vi "ziModSetVector.vi"(8 "error in":errorcluster, 9 "VectorWave In":T2, 10 "Path":string, 11 "ModHandle In":T1 {"ModHandle" format="0x%08x"; "Conn" format="0x%08x"}) -> (0 "error out":errorcluster, 3 "ModHandle Out":T1 {"ModHandle" format="0x%08x"; "Conn" format="0x%08x"})   [LabVIEW 2009, in "Zurich Instruments LabOne.lvlib"]
uses:
  <instrlib>/Zurich Instruments LabOne/Zurich Instruments LabOne.lvlib
  <instrlib>/Zurich Instruments LabOne/Public/Data/ziTypeCoreVectorWave.ctl
  <instrlib>/Zurich Instruments LabOne/Public/Modules/ziTypeModHandle.ctl
  <instrlib>/Zurich Instruments LabOne/Private/ziLV32.dll
panel:
  out "VectorWave Out":T2
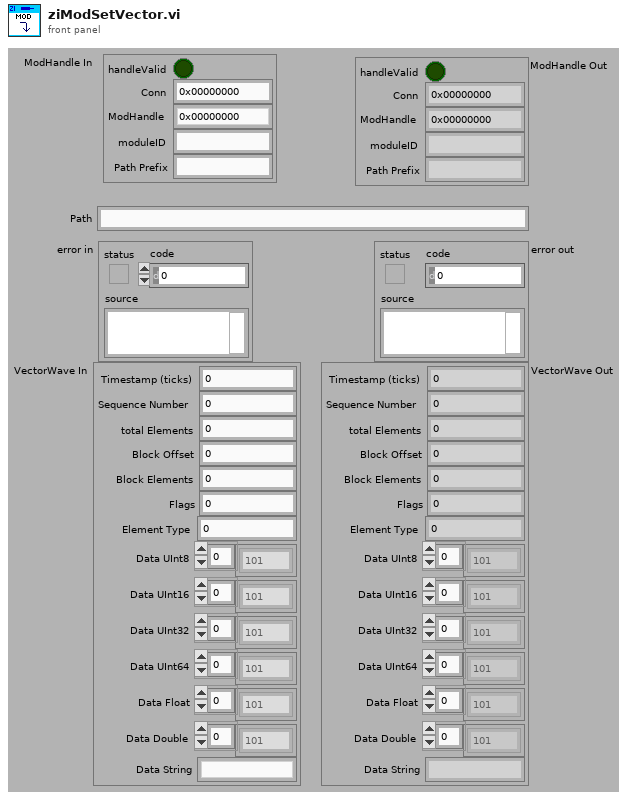
[diagram p1: front panel]
types:
  T1 = typedef "Zurich Instruments LabOne.lvlib/ziTypeModHandle.ctl" = cluster{"handleValid":bool, "Conn":u64, "ModHandle":u64, "moduleID":string, "Path Prefix":string}
  T2 = typedef "Zurich Instruments LabOne.lvlib/ziTypeCoreVectorWave.ctl" = cluster{"Timestamp (ticks)":u64, "Sequence Number":u32, "total Elements":u64, "Block Offset":u64, "Block Elements":u32, "Flags":u8, "Element Type":u8, "Data UInt8":u8[], "Data UInt16":u16[], "Data UInt32":u32[], "Data UInt64":u64[], "Data Float":sgl[], "Data Double":dbl[], "Data String":string}
  T3 = enum8{"Unit8", "Unit16", "Unit32", "Unit64", "Float", "Double", "ASCII", "NA"}
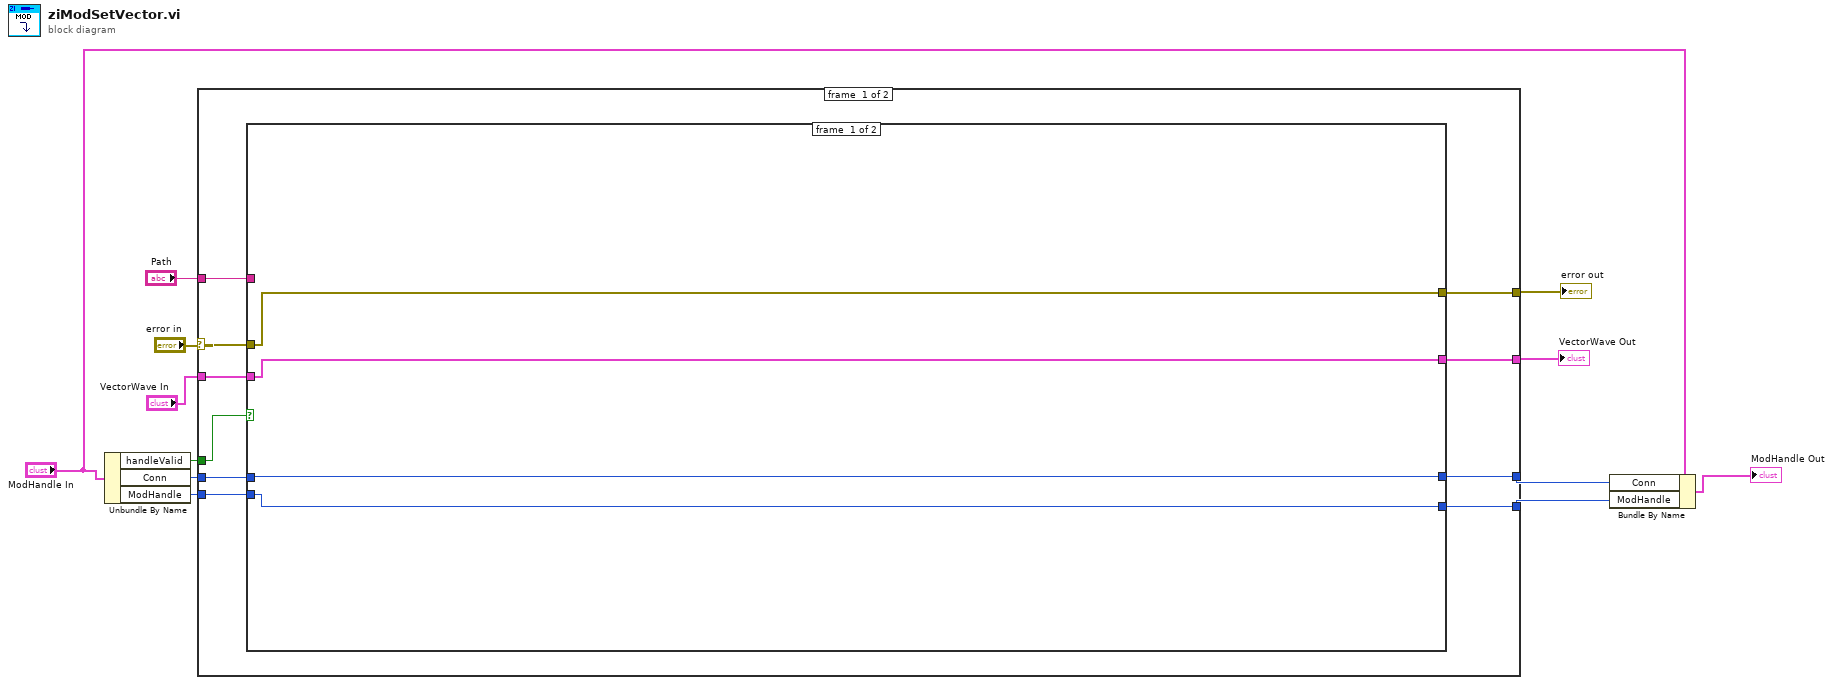
[diagram p0: block diagram]
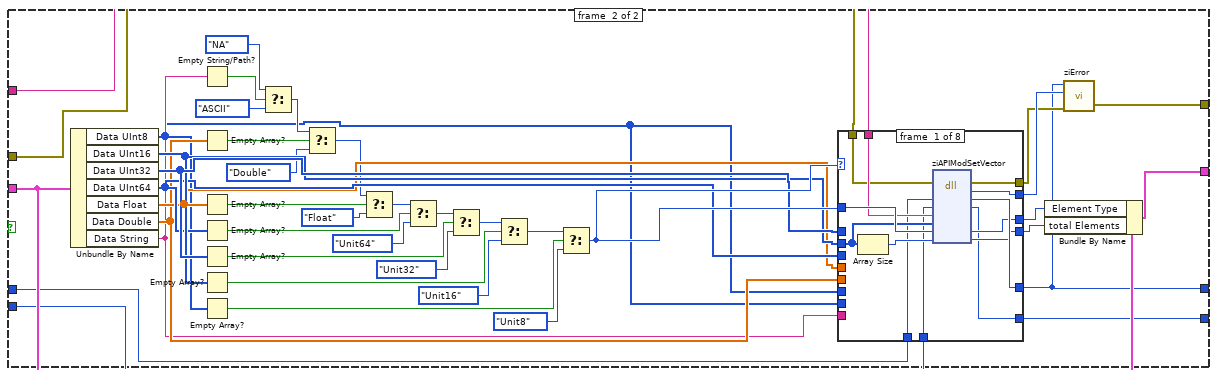
[diagram p2: hidden frame]
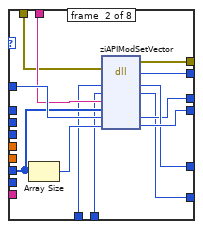
[diagram p3: hidden frame]
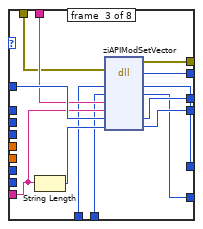
[diagram p4: hidden frame]
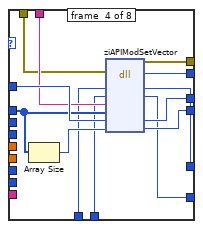
[diagram p5: hidden frame]
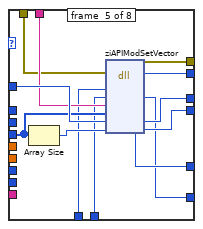
[diagram p6: hidden frame]
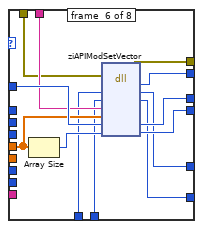
[diagram p7: hidden frame]
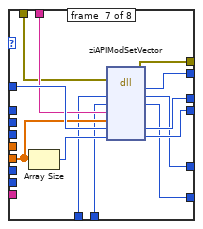
[diagram p8: hidden frame]
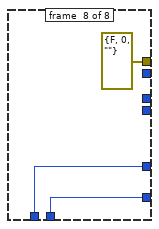
[diagram p9: hidden frame]
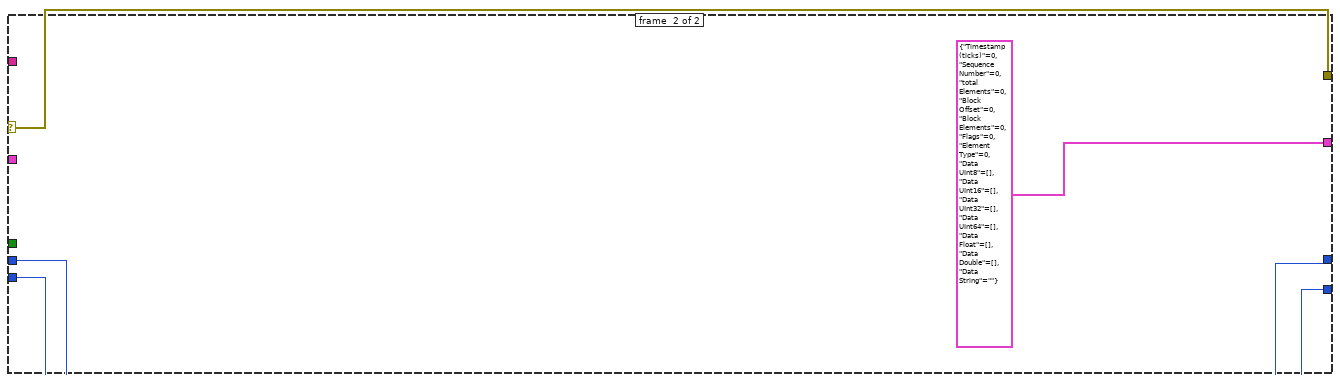
[diagram p10: hidden frame]
diagram:
  n1 = Unbundle By Name("ModHandle In") -> ("handleValid"=w3:bool, "Conn"=w7:u64, "ModHandle"=w6:u64)
  n2 = case shown="No Error" "error in" {
    selector: "error in" -> [w16 w166]
    tunnel: [w22 w166] -> w12
    tunnel: "Path" -> [w19 _]
    tunnel: "VectorWave In" -> [w21 _]
    tunnel: [w20 T2 {"Timestamp (ticks)"=0, "Sequence Number"=0, "total Elements"=0, "Block Offset"=0, "Block Elements"=0, "Flags"=0, "Element Type"=0, "Data UInt8"=[], "Data UInt16"=[], "Data UInt32"=[], "Data UInt64"=[], "Data Float"=[], "Data Double"=[], "Data String"=""} ("VectorWave In")] -> w9
    tunnel: w7 -> [w18 w163]
    tunnel: w6 -> [w17 w164]
    tunnel: [w15 w163] -> w5
    tunnel: [w14 w164] -> w4
    tunnel: w3 -> [w13 _]
    frame #0 {
      n3 = case shown="True" w13 {
        tunnel: [w26 w68] -> w22
        tunnel: w21 -> [w25 w58]
        tunnel: [w25 w57] -> w20
        tunnel: w19 -> [_ w32]
        tunnel: w18 -> [w24 w31]
        tunnel: w17 -> [w23 w30]
        tunnel: w16 -> [w26 w29]
        tunnel: [w24 w28] -> w15
        tunnel: [w23 w27] -> w14
        frame #0 {
        }
        frame #1 {
          n4 = Unbundle By Name(w58) -> ("Data UInt8"=w33:u8[], "Data UInt16"=w52:u16[], "Data UInt32"=w53:u32[], "Data UInt64"=w51:u64[], "Data Float"=w50:sgl[], "Data Double"=w49:dbl[], "Data String"=w48:string)
          n5 = Empty String/Path?(string/path=w48) -> (empty?=w67:bool)
          n6 = Empty Array?(array=w49) -> (empty?=w66:bool)
          n7 = Empty Array?(array=w50) -> (empty?=w65:bool)
          n8 = Empty Array?(array=w51) -> (empty?=w64:bool)
          n9 = Empty Array?(array=w53) -> (empty?=w63:bool)
          n10 = Empty Array?(array=w52) -> (empty?=w62:bool)
          n11 = Empty Array?(array=w33) -> (empty?=w61:bool)
          n12 = Select(t=T3."NA", s=w67, f=T3."ASCII") -> (s? t:f=w34:T3)
          n13 = Select(t=w34, s=w66, f=T3."Double") -> (s? t:f=w35:T3)
          n14 = Select(t=w35, s=w65, f=T3."Float") -> (s? t:f=w36:T3)
          n15 = Select(t=w36, s=w64, f=T3."Unit64") -> (s? t:f=w37:T3)
          n16 = Select(t=w37, s=w63, f=T3."Unit32") -> (s? t:f=w38:T3)
          n17 = Select(t=w38, s=w62, f=T3."Unit16") -> (s? t:f=w39:T3)
          n18 = Select(t=w39, s=w61, f=T3."Unit8") -> (s? t:f=w54:T3)
          n19 = case shown="\"NA\", Default" w54 {
            tunnel: [w81 w89 w101 w114 w127 w140 w153 _] -> w60
            tunnel: [w80 w90 w102 w115 w128 w141 w154 errorcluster {"status"=FALSE, "code"=0, "source"=""} ("error out")] -> w59
            tunnel: [w79 w88 w100 w113 w126 w139 w152 w161] -> w28
            tunnel: w54 -> [w77 w93 w106 w119 w133 w146 w159 _]
            tunnel: [w76 w86 w103 w116 w129 w142 w155 _] -> w56
            tunnel: [w75 w91 w104 w117 w130 w143 w156 _] -> w55
            tunnel: w53 -> [_ _ _ w118 _ _ _ _]
            tunnel: w52 -> [w74 _ _ _ _ _ _ _]
            tunnel: w51 -> [_ _ _ _ w131 _ _ _]
            tunnel: w50 -> [_ _ _ _ _ w144 _ _]
            tunnel: w49 -> [_ _ _ _ _ _ w157 _]
            tunnel: w48 -> [_ _ w105 _ _ _ _ _]
            tunnel: w33 -> [_ _ _ _ _ _ _ _]
            tunnel: w33 -> [_ w92 _ _ _ _ _ _]
            tunnel: w32 -> [w73 w87 w99 w112 w125 w138 w151 _]
            tunnel: w31 -> [w72 w85 w98 w110 w123 w136 w149 w161]
            tunnel: w30 -> [w71 w84 w97 w111 w124 w137 w150 w160]
            tunnel: w29 -> [w70 w83 w96 w109 w122 w135 w148 _]
            tunnel: [w69 w82 w95 w108 w121 w134 w147 w160] -> w27
            frame #0 {
              n20 = Array Size(array=w74) -> (size(s)=w78:i32)
              n21 = dll-call lib="C:/Program Files (x86)/National Instruments/LabVIEW 2009/instr.lib/Zurich Instruments LabOne/Private/ziLV*.*" fn="ziAPIModSetVector"(error in=w70, "Conn"=w72, "ModHandle"=w71, "Path"=w73, "Pointer"=w74, "vectorElementType"=w77, "vectorSizeElements"=w78) -> (error out=w80:errorcluster, "return type"=w81:u8, "Conn"=w79:u64, "ModHandle"=w69:u64, "vectorElementType"=w76:u8, "vectorSizeElements"=w75:u64)  [unwired: 2 in, 3 out]
            }
            frame #1 {
              n22 = Array Size(array=w92) -> (size(s)=w94:i32)
              n23 = dll-call lib="C:/Program Files (x86)/National Instruments/LabVIEW 2009/instr.lib/Zurich Instruments LabOne/Private/ziLV*.*" fn="ziAPIModSetVector"(error in=w83, "Conn"=w85, "ModHandle"=w84, "Path"=w87, "Pointer"=w92, "vectorElementType"=w93, "vectorSizeElements"=w94) -> (error out=w90:errorcluster, "return type"=w89:u8, "Conn"=w88:u64, "ModHandle"=w82:u64, "vectorElementType"=w86:u8, "vectorSizeElements"=w91:u64)  [unwired: 2 in, 3 out]
            }
            frame #2 {
              n24 = String Length(string=w105) -> (length=w107:i32)
              n25 = dll-call lib="C:/Program Files (x86)/National Instruments/LabVIEW 2009/instr.lib/Zurich Instruments LabOne/Private/ziLV*.*" fn="ziAPIModSetVector"(error in=w96, "Conn"=w98, "ModHandle"=w97, "Path"=w99, "Pointer"=w105, "vectorElementType"=w106, "vectorSizeElements"=w107) -> (error out=w102:errorcluster, "return type"=w101:u8, "Conn"=w100:u64, "ModHandle"=w95:u64, "vectorElementType"=w103:u8, "vectorSizeElements"=w104:u64)  [unwired: 2 in, 3 out]
            }
            frame #3 {
              n26 = Array Size(array=w118) -> (size(s)=w120:i32)
              n27 = dll-call lib="C:/Program Files (x86)/National Instruments/LabVIEW 2009/instr.lib/Zurich Instruments LabOne/Private/ziLV*.*" fn="ziAPIModSetVector"(error in=w109, "Conn"=w110, "ModHandle"=w111, "Path"=w112, "Pointer"=w118, "vectorElementType"=w119, "vectorSizeElements"=w120) -> (error out=w115:errorcluster, "return type"=w114:u8, "Conn"=w113:u64, "ModHandle"=w108:u64, "vectorElementType"=w116:u8, "vectorSizeElements"=w117:u64)  [unwired: 2 in, 3 out]
            }
            frame #4 {
              n28 = Array Size(array=w131) -> (size(s)=w132:i32)
              n29 = dll-call lib="C:/Program Files (x86)/National Instruments/LabVIEW 2009/instr.lib/Zurich Instruments LabOne/Private/ziLV*.*" fn="ziAPIModSetVector"(error in=w122, "Conn"=w123, "ModHandle"=w124, "Path"=w125, "Pointer"=w131, "vectorElementType"=w133, "vectorSizeElements"=w132) -> (error out=w128:errorcluster, "return type"=w127:u8, "Conn"=w126:u64, "ModHandle"=w121:u64, "vectorElementType"=w129:u8, "vectorSizeElements"=w130:u64)  [unwired: 2 in, 3 out]
            }
            frame #5 {
              n30 = Array Size(array=w144) -> (size(s)=w145:i32)
              n31 = dll-call lib="C:/Program Files (x86)/National Instruments/LabVIEW 2009/instr.lib/Zurich Instruments LabOne/Private/ziLV*.*" fn="ziAPIModSetVector"(error in=w135, "Conn"=w136, "ModHandle"=w137, "Path"=w138, "Pointer"=w144, "vectorElementType"=w146, "vectorSizeElements"=w145) -> (error out=w141:errorcluster, "return type"=w140:u8, "Conn"=w139:u64, "ModHandle"=w134:u64, "vectorElementType"=w142:u8, "vectorSizeElements"=w143:u64)  [unwired: 2 in, 3 out]
            }
            frame #6 {
              n32 = Array Size(array=w157) -> (size(s)=w158:i32)
              n33 = dll-call lib="C:/Program Files (x86)/National Instruments/LabVIEW 2009/instr.lib/Zurich Instruments LabOne/Private/ziLV*.*" fn="ziAPIModSetVector"(error in=w148, "Conn"=w149, "ModHandle"=w150, "Path"=w151, "Pointer"=w157, "vectorElementType"=w159, "vectorSizeElements"=w158) -> (error out=w154:errorcluster, "return type"=w153:u8, "Conn"=w152:u64, "ModHandle"=w147:u64, "vectorElementType"=w155:u8, "vectorSizeElements"=w156:u64)  [unwired: 2 in, 3 out]
            }
            frame #7 {
            }
          }
          n34 = Bundle By Name(cluster=w58, "Element Type"=w56, "total Elements"=w55) -> (w57:T2)
          n35 = call <instrlib>:"ziError.vi"("Conn"=w28, "ziErrorCode"=w60, "Error In"=w59) -> ("Error Out"=w68:errorcluster)  [unwired: 2 in, 1 out]
        }
      }
    }
    frame #1 {
    }
  }
  "error out" <- w12
  "VectorWave Out" <- w9
  n36 = Bundle By Name(cluster="ModHandle In", "Conn"=w5, "ModHandle"=w4) -> (→"ModHandle Out":T1)
